vi "UHR-Fleezers Control (host) - Lorentz v5.vi"() -> ()   [LabVIEW 2014] (continued)
                n1783 = Number To Decimal String(number="Flush rate (uL/m)") -> (decimal integer string=w2729:string)  [unwired: 1 in]
                n1784 = Concatenate Strings("irate  " ("string"), w2729, " u/m" ("string"), "\r") -> (w2731:string)
                n1785 = VISA Write(VISA resource name=w2733, write buffer=w2731) -> (VISA resource name out=w2727:refnum<visa-resource-name>)  [unwired: 1 in, 2 out]
                n1786 = Reciprocal(x="Flush rate (uL/m)") -> (1/x=w2712:dbl)
                n1787 = Number To Decimal String(number="Volume (uL)") -> (decimal integer string=w2718:string)  [unwired: 1 in]
                n1788 = Multiply(x="Volume (uL)", y=w2712) -> (x*y=w2711:dbl)
                n1789 = Concatenate Strings("tvolume  " ("string"), w2718, " u" ("string"), "\r") -> (w2716:string)
                n1790 = Multiply(x=w2711, y=60000.0) -> (x*y=w2709:dbl)
                n1791 = VISA Write(VISA resource name=w2727, write buffer=w2716) -> (VISA resource name out=w2715:refnum<visa-resource-name>)  [unwired: 1 in, 2 out]
                n1792 = Concatenate Strings("cvolume" ("string"), "\r") -> (w2714:string)
                n1793 = VISA Write(VISA resource name=w2715, write buffer=w2714) -> (VISA resource name out=w2725:refnum<visa-resource-name>)  [unwired: 1 in, 2 out]
                n1794 = Concatenate Strings("irun" ("string"), "\r") -> (w2723:string)
                n1795 = VISA Write(VISA resource name=w2725, write buffer=w2723) -> (VISA resource name out=w2713:refnum<visa-resource-name>)  [unwired: 1 in, 2 out]
              }
              frame #1 {
                # "Have to wait until\nflow is done to reset\nrate"
                n1796 = Add(x=w2736, y=100.0) -> (x+y=w2735:dbl)
                n1797 = Wait (ms)(milliseconds to wait=w2735) -> ()  [unwired: 1 out]
              }
              frame #2 {
                # "reset flow rate to usual flow rate"
                n1798 = local read "Flow rate (uL/h)"() -> (w2748:dbl)
                n1799 = Number To Decimal String(number=w2748) -> (decimal integer string=w2746:string)  [unwired: 1 in]
                n1800 = Concatenate Strings("irate  " ("string"), w2746, " u/h" ("string"), "\r") -> (w2744:string)
                n1801 = VISA Write(VISA resource name=w2742, write buffer=w2744) -> (VISA resource name out=w2738:refnum<visa-resource-name>)  [unwired: 1 in, 2 out]
                n1802 = Concatenate Strings("cvolume" ("string"), "\r") -> (w2739:string)
                n1803 = VISA Write(VISA resource name=w2738, write buffer=w2739) -> ()  [unwired: 1 in, 3 out]
              }
            }
            n1804 = local read "Save Event Log?"() -> (w2688:bool)
            n1805 = local read "Saving..."() -> (w2687:bool)
            n1806 = And(x=w2688, y=w2687) -> (x .and. y?=w2689:bool)
            n1807 = case shown="True" w2689 {
              tunnel: w2691 -> [_ w2698]
              tunnel: w2690 -> [_ w2697]
              frame False {
              }
              frame True {
                n1808 = Number To Decimal String(number=w2698) -> (decimal integer string=w2702:string)  [unwired: 1 in]
                n1809 = Number To Decimal String(number=w2697) -> (decimal integer string=w2704:string)  [unwired: 1 in]
                n1810 = local read "log file ref"() -> (w2699:refnum<file>)
                n1811 = local read "Time (s)"() -> (w2700:dbl)
                n1812 = Concatenate Strings("pump 2 flushing ", w2702, " uL at ", w2704, " ul/min") -> (w2706:string)
                n1813 = call "write to event log.vi"("log file ref"=w2699, "time"=w2700, "input string"=w2706) -> ()  [unwired: 8 in]
              }
            }
          }
          frame Enabled {
          }
        }
      }
      event "Flush Pump 3": Value Change {
        n1814 = event-data() -> ()  [unwired: 7 out]
        n1815 = disable-structure shown="Disabled" {
          disable-tunnel: ["Flush Pump 3" _] -> w2750
          disable-tunnel: w2749 -> [w2756 _]
          frame Disabled {
            n1816 = flat-sequence {
              tunnel: w2756 -> [w2771]
              tunnel: ["Flush rate (uL/m) P3"] -> w2752
              tunnel: ["Volume (uL) P3"] -> w2751
              frame #0 {
                # "set paramaters (rate, volume) for flush, clear volume"
                n1817 = Number To Decimal String(number="Flush rate (uL/m) P3") -> (decimal integer string=w2791:string)  [unwired: 1 in]
                n1818 = local write "Inject Pump 3"(TRUE ("Inject Pump 3")) -> ()
                n1819 = Concatenate Strings("irate  " ("string"), w2791, " u/m" ("string"), "\r") -> (w2793:string)
                n1820 = VISA Write(VISA resource name=w2771, write buffer=w2793) -> (VISA resource name out=w2789:refnum<visa-resource-name>)  [unwired: 1 in, 2 out]
                n1821 = Reciprocal(x="Flush rate (uL/m) P3") -> (1/x=w2775:dbl)
                n1822 = Number To Decimal String(number="Volume (uL) P3") -> (decimal integer string=w2780:string)  [unwired: 1 in]
                n1823 = Multiply(x="Volume (uL) P3", y=w2775) -> (x*y=w2774:dbl)
                n1824 = Concatenate Strings("tvolume  " ("string"), w2780, " u" ("string"), "\r") -> (w2778:string)
                n1825 = Multiply(x=w2774, y=60.0) -> (x*y=→"HP3 Flush Time (s)":dbl)
                n1826 = VISA Write(VISA resource name=w2789, write buffer=w2778) -> (VISA resource name out=w2777:refnum<visa-resource-name>)  [unwired: 1 in, 2 out]
                n1827 = Concatenate Strings("cvolume" ("string"), "\r") -> (w2776:string)
                n1828 = VISA Write(VISA resource name=w2777, write buffer=w2776) -> (VISA resource name out=w2787:refnum<visa-resource-name>)  [unwired: 1 in, 2 out]
                n1829 = Concatenate Strings("irun" ("string"), "\r") -> (w2785:string)
                n1830 = VISA Write(VISA resource name=w2787, write buffer=w2785) -> ()  [unwired: 1 in, 3 out]
              }
              frame #1 {
                "Flushing P3" <- TRUE ("Flushing P3")
              }
            }
            n1831 = local read "Save Event Log?"() -> (w2754:bool)
            n1832 = local read "Saving..."() -> (w2755:bool)
            n1833 = And(x=w2754, y=w2755) -> (x .and. y?=w2753:bool)
            n1834 = case shown="True" w2753 {
              tunnel: w2752 -> [_ w2759]
              tunnel: w2751 -> [_ w2758]
              frame False {
              }
              frame True {
                n1835 = Number To Decimal String(number=w2758) -> (decimal integer string=w2763:string)  [unwired: 1 in]
                n1836 = Number To Decimal String(number=w2759) -> (decimal integer string=w2765:string)  [unwired: 1 in]
                n1837 = local read "log file ref"() -> (w2760:refnum<file>)
                n1838 = local read "Time (s)"() -> (w2761:dbl)
                n1839 = Concatenate Strings("pump 3 flushing ", w2763, " uL at ", w2765, " ul/min") -> (w2767:string)
                n1840 = call "write to event log.vi"("log file ref"=w2760, "time"=w2761, "input string"=w2767) -> ()  [unwired: 8 in]
              }
            }
          }
          frame Enabled {
          }
        }
      }
      event "Flush Pump 1": Value Change {
        n1841 = event-data() -> ()  [unwired: 7 out]
        n1842 = disable-structure shown="Disabled" {
          disable-tunnel: ["Flush Pump 1" _] -> w2797
          disable-tunnel: w2796 -> [w2803 _]
          frame Disabled {
            n1843 = flat-sequence {
              tunnel: [w2824] -> w2805
              tunnel: w2803 -> [w2819]
              tunnel: ["Volume (uL) P1"] -> w2799
              tunnel: ["Flush rate (uL/m) P1"] -> w2798
              tunnel: w2805 -> [_]
              frame #0 {
                # "set paramaters (rate, volume) for flush, clear volume"
                n1844 = local write "Inject Pump 1"(TRUE ("Inject Pump 1")) -> ()
                n1845 = Number To Decimal String(number="Flush rate (uL/m) P1") -> (decimal integer string=w2840:string)  [unwired: 1 in]
                n1846 = Concatenate Strings("irate  " ("string"), w2840, " u/m" ("string"), "\r") -> (w2842:string)
                n1847 = VISA Write(VISA resource name=w2819, write buffer=w2842) -> (VISA resource name out=w2838:refnum<visa-resource-name>)  [unwired: 1 in, 2 out]
                n1848 = Reciprocal(x="Flush rate (uL/m) P1") -> (1/x=w2823:dbl)
                n1849 = Number To Decimal String(number="Volume (uL) P1") -> (decimal integer string=w2829:string)  [unwired: 1 in]
                n1850 = Multiply(x="Volume (uL) P1", y=w2823) -> (x*y=w2822:dbl)
                n1851 = Concatenate Strings("tvolume  " ("string"), w2829, " u" ("string"), "\r") -> (w2827:string)
                n1852 = Multiply(x=w2822, y=60.0) -> (x*y=→"HP1 Flush Time (s)":dbl)
                n1853 = VISA Write(VISA resource name=w2838, write buffer=w2827) -> (VISA resource name out=w2826:refnum<visa-resource-name>)  [unwired: 1 in, 2 out]
                n1854 = Concatenate Strings("cvolume" ("string"), "\r") -> (w2825:string)
                n1855 = VISA Write(VISA resource name=w2826, write buffer=w2825) -> (VISA resource name out=w2836:refnum<visa-resource-name>)  [unwired: 1 in, 2 out]
                n1856 = Concatenate Strings("irun" ("string"), "\r") -> (w2834:string)
                n1857 = VISA Write(VISA resource name=w2836, write buffer=w2834) -> (VISA resource name out=w2824:refnum<visa-resource-name>)  [unwired: 1 in, 2 out]
              }
              frame #1 {
                "Flushing P1" <- TRUE ("Flushing P3")
              }
            }
            n1858 = local read "Saving..."() -> (w2800:bool)
            n1859 = local read "Save Event Log?"() -> (w2801:bool)
            n1860 = And(x=w2801, y=w2800) -> (x .and. y?=w2802:bool)
            n1861 = case shown="True" w2802 {
              tunnel: w2799 -> [_ w2808]
              tunnel: w2798 -> [_ w2807]
              frame False {
              }
              frame True {
                n1862 = Number To Decimal String(number=w2808) -> (decimal integer string=w2812:string)  [unwired: 1 in]
                n1863 = Number To Decimal String(number=w2807) -> (decimal integer string=w2810:string)  [unwired: 1 in]
                n1864 = local read "log file ref"() -> (w2814:refnum<file>)
                n1865 = local read "Time (s)"() -> (w2815:dbl)
                n1866 = Concatenate Strings("pump 1 flushing ", w2812, " uL at ", w2810, " ul/min") -> (w2806:string)
                n1867 = call "write to event log.vi"("log file ref"=w2814, "time"=w2815, "input string"=w2806) -> ()  [unwired: 8 in]
              }
            }
          }
          frame Enabled {
          }
        }
      }
      event "Clear Volume": Value Change {
        n1868 = event-data() -> ()  [unwired: 7 out]
        n1869 = disable-structure shown="Disabled" {
          disable-tunnel: ["Clear Volume" _] -> w2846
          disable-tunnel: w2845 -> [w2847 _]
          frame Disabled {
            n1870 = Concatenate Strings("cvolume" ("string"), "\r") -> (w2848:string)
            n1871 = VISA Write(VISA resource name=w2847, write buffer=w2848) -> ()  [unwired: 1 in, 3 out]
          }
          frame Enabled {
          }
        }
      }
      event "Clear Volume P3": Value Change {
        n1872 = event-data() -> ()  [unwired: 7 out]
        n1873 = disable-structure shown="Disabled" {
          disable-tunnel: w2852 -> [w2854 _]
          frame Disabled {
            n1874 = Concatenate Strings("cvolume" ("string"), "\r") -> (w2855:string)
            n1875 = VISA Write(VISA resource name=w2854, write buffer=w2855) -> ()  [unwired: 1 in, 3 out]
            n1876 = local write "Clear Volume P3"(FALSE ("Clear Volume P3")) -> ()
          }
          frame Enabled {
          }
        }
      }
      event "Clear Volume P1": Value Change {
        n1877 = event-data() -> ()  [unwired: 7 out]
        n1878 = disable-structure shown="Disabled" {
          disable-tunnel: w2858 -> [w2860 _]
          frame Disabled {
            n1879 = Concatenate Strings("cvolume" ("string"), "\r") -> (w2861:string)
            n1880 = local write "Clear Volume P1"(FALSE ("Clear Volume P1")) -> ()
            n1881 = VISA Write(VISA resource name=w2860, write buffer=w2861) -> ()  [unwired: 1 in, 3 out]
          }
          frame Enabled {
          }
        }
      }
      event "Display On P3": Value Change {
        n1882 = event-data() -> ()  [unwired: 7 out]
        n1883 = disable-structure shown="Disabled" {
          disable-tunnel: w2864 -> [w2865 _]
          frame Disabled {
            n1884 = Select(t="dim 100", s="Display On P3", f="dim 0") -> (s? t:f=w2868:string)
            n1885 = Concatenate Strings(w2868, "\r") -> (w2870:string)
            n1886 = VISA Write(VISA resource name=w2865, write buffer=w2870) -> ()  [unwired: 1 in, 3 out]
          }
          frame Enabled {
          }
        }
      }
      event "Display On P1": Value Change {
        n1887 = event-data() -> ()  [unwired: 7 out]
        n1888 = disable-structure shown="Disabled" {
          disable-tunnel: w2872 -> [w2873 _]
          frame Disabled {
            n1889 = Select(t="dim 100", s="Display On P1", f="dim 0") -> (s? t:f=w2876:string)
            n1890 = Concatenate Strings(w2876, "\r") -> (w2878:string)
            n1891 = VISA Write(VISA resource name=w2873, write buffer=w2878) -> ()  [unwired: 1 in, 3 out]
          }
          frame Enabled {
          }
        }
      }
      event "Retract Pump 3": Value Change {
        n1892 = event-data() -> ()  [unwired: 7 out]
        n1893 = disable-structure shown="Disabled" {
          disable-tunnel: w2880 -> [w2881 _]
          frame Disabled {
            n1894 = local write "Retract Pump 3"(FALSE ("Retract Pump 3")) -> ()
            n1895 = case shown="True" "Retract Pump 3" {
              tunnel: w2881 -> [_ w2884]
              frame False {
              }
              frame True {
                n1896 = Number To Decimal String(number="Retract Rate (uL/m)") -> (decimal integer string=w2902:string)  [unwired: 1 in]
                n1897 = Concatenate Strings("wrate  " ("string"), w2902, " u/m" ("string"), "\r") -> (w2904:string)
                n1898 = VISA Write(VISA resource name=w2884, write buffer=w2904) -> (VISA resource name out=w2895:refnum<visa-resource-name>)  [unwired: 1 in, 2 out]
                n1899 = Number To Decimal String(number="Retract Vol 3 (uL)") -> (decimal integer string=w2897:string)  [unwired: 1 in]
                n1900 = Concatenate Strings("tvolume  " ("string"), w2897, " u" ("string"), "\r") -> (w2894:string)
                n1901 = VISA Write(VISA resource name=w2895, write buffer=w2894) -> (VISA resource name out=w2890:refnum<visa-resource-name>)  [unwired: 1 in, 2 out]
                n1902 = Concatenate Strings("cvolume" ("string"), "\r") -> (w2891:string)
                n1903 = VISA Write(VISA resource name=w2890, write buffer=w2891) -> (VISA resource name out=w2885:refnum<visa-resource-name>)  [unwired: 1 in, 2 out]
                n1904 = Concatenate Strings("wrun" ("string"), "\r") -> (w2886:string)
                n1905 = VISA Write(VISA resource name=w2885, write buffer=w2886) -> ()  [unwired: 1 in, 3 out]
              }
            }
          }
          frame Enabled {
          }
        }
      }
      event "Retract Pump 1": Value Change {
        n1906 = event-data() -> ()  [unwired: 7 out]
        n1907 = disable-structure shown="Disabled" {
          disable-tunnel: w2906 -> [w2907 _]
          frame Disabled {
            n1908 = local write "Retract Pump 1"(FALSE ("Retract Pump 1")) -> ()
            n1909 = case shown="True" "Retract Pump 1" {
              tunnel: w2907 -> [_ w2912]
              frame False {
              }
              frame True {
                n1910 = local read "Retract Rate (uL/m)"() -> (w2910:dbl)
                n1911 = Number To Decimal String(number=w2910) -> (decimal integer string=w2928:string)  [unwired: 1 in]
                n1912 = Concatenate Strings("wrate  " ("string"), w2928, " u/m" ("string"), "\r") -> (w2930:string)
                n1913 = VISA Write(VISA resource name=w2912, write buffer=w2930) -> (VISA resource name out=w2922:refnum<visa-resource-name>)  [unwired: 1 in, 2 out]
                n1914 = Number To Decimal String(number="Retract Vol 1 (uL)") -> (decimal integer string=w2924:string)  [unwired: 1 in]
                n1915 = Concatenate Strings("tvolume  " ("string"), w2924, " u" ("string"), "\r") -> (w2921:string)
                n1916 = VISA Write(VISA resource name=w2922, write buffer=w2921) -> (VISA resource name out=w2918:refnum<visa-resource-name>)  [unwired: 1 in, 2 out]
                n1917 = Concatenate Strings("cvolume" ("string"), "\r") -> (w2919:string)
                n1918 = VISA Write(VISA resource name=w2918, write buffer=w2919) -> (VISA resource name out=w2913:refnum<visa-resource-name>)  [unwired: 1 in, 2 out]
                n1919 = Concatenate Strings("wrun" ("string"), "\r") -> (w2914:string)
                n1920 = VISA Write(VISA resource name=w2913, write buffer=w2914) -> ()  [unwired: 1 in, 3 out]
              }
            }
          }
          frame Enabled {
          }
        }
      }
      event "Flip Green Filter": Value Change {
        n1921 = event-data() -> ()  [unwired: 7 out]
        n1922 = Not(x="Flip Green Filter") -> (.not. x?=w2933:bool)
        n1923 = local write "Flip Green Filter"(w2933) -> ()
        n1924 = flat-sequence {
          tunnel: [w2942] -> w2938
          tunnel: [w2941] -> w2937
          tunnel: w2932 -> [w2940]
          tunnel: [w2945] -> w2936
          tunnel: w2938 -> [w2945]
          tunnel: [w2944] -> w2935
          tunnel: w2937 -> [w2944]
          tunnel: w2936 -> [w2949]
          tunnel: w2935 -> [w2948]
          tunnel: [w2947] -> w2939
          frame #0 {
            n1925 = xnode "Read/Write Control"("FPGA VI Reference In"=w2940, "Green Filter Flipper"=TRUE) -> ("FPGA VI Reference Out"=w2942:T35, "error out"=w2941:errorcluster)  [unwired: 1 in]
          }
          frame #1 {
            n1926 = Wait (ms)(milliseconds to wait=u32 100) -> ()  [unwired: 1 out]
          }
          frame #2 {
            n1927 = xnode "Read/Write Control"("FPGA VI Reference In"=w2949, "error in"=w2948, "Green Filter Flipper"=FALSE) -> ("error out"=w2947:errorcluster)  [unwired: 1 out]
          }
        }
      }
      event "Pump 1 contents", "Pump 3 contents": Value Change {
        n1928 = event-data() -> ()  [unwired: 7 out]
        n1929 = local read "Pump 1 contents"() -> (→"Pump 1 cont disp":string)
        n1930 = local read "Pump 3 contents"() -> (→"Pump 3 cont disp":string)
      }
      event "Reset Trap Pos. FB": Value Change {
        n1931 = event-data() -> ()  [unwired: 7 out]
        n1932 = xnode "Read/Write Control"("FPGA VI Reference In"=w2953, "Trap Pos. FB Reset"="Reset Trap Pos. FB") -> ()  [unwired: 1 in, 2 out]
      }
      event "Rem fb disp offset": Value Change {
        n1933 = event-data() -> ()  [unwired: 7 out]
        n1934 = local write "Rem fb disp offset"(FALSE ("Rem fb disp offset")) -> ()
        n1935 = local read "Mean Trap Positions (nm)"() -> (w2956:T4)
        n1936 = local read "FB Trap Pos Offset"() -> (w2958:dbl)
        n1937 = Unbundle By Name(w2956) -> ("T1 X"=w2955:dbl)
        n1938 = Subtract(x=w2958, y=w2955) -> (x-y=w2957:dbl)
        n1939 = local write "FB Trap Pos Offset"(w2957) -> ()
      }
      event "Threshold (nm)": Value Change {
        n1940 = event-data() -> ()  [unwired: 7 out]
        n1941 = flat-sequence {
          tunnel: [w2963] -> w2961
          tunnel: w2960 -> [w2962]
          tunnel: w2961 -> [w2974]
          frame #0 {
            n1942 = xnode "Read/Write Control"("FPGA VI Reference In"=w2962) -> ("FPGA VI Reference Out"=w2966:T35, "error out"=w2965:errorcluster, "FPGA TTrig Thresh"=w2967:i64)  [unwired: 1 in]
            n1943 = local read "Threshold stored (nm)"() -> (w2973:dbl)
            n1944 = local read "Threshold (nm)"() -> (w2963:dbl)
            n1945 = local read "AOM X Cal (nm/MHz)"() -> (w2971:dbl)
            n1946 = Subtract(x=w2963, y=w2973) -> (x-y=w2972:dbl)
            n1947 = Divide(x=w2972, y=w2971) -> (x/y=w2969:dbl)
            n1948 = call "IR AOM freq to word.vi"("Frequency In (MHz)"=w2969) -> ("Frequency Word Out (double)"=w2970:dbl)
            n1949 = To Quad Integer(1:w2970) -> (0:w2968:i64)
            n1950 = Add(x=w2967, y=w2968) -> (x+y=w2964:i64)
            n1951 = xnode "Read/Write Control"("FPGA VI Reference In"=w2966, "error in"=w2965, "FPGA TTrig Thresh"=w2964) -> ()  [unwired: 2 out]
          }
          frame #1 {
            "Threshold stored (nm)" <- w2974
          }
        }
      }
      event "FB Trig Integrate": Value Change {
        n1952 = event-data() -> ()  [unwired: 7 out]
        n1953 = local read "FB Trig Integrate"() -> (w2977:u32)
        n1954 = xnode "Read/Write Control"("FPGA VI Reference In"=w2975, "FB Trig Integrate"=w2977) -> ("error out"=w2976:errorcluster)  [unwired: 1 in, 1 out]
      }
      event "11": Value Change {
        n1955 = event-data() -> ()  [unwired: 7 out]
        n1956 = local read "11"() -> (w2978:bool)
        n1957 = case shown="True" w2978 {
          frame False {
          }
          frame True {
            n1958 = local read "Messages"() -> (w2980:string)
            n1959 = call "Update messages.vi"("Message to add"="You kicked it up to 11!", "Old message string"=w2980) -> ("New message string"=w2981:string)
            n1960 = call <vilib>:"Beep.vi"() -> ()  [unwired: 12 in]
            n1961 = local write "Messages"(w2981) -> ()
          }
        }
      }
      event "Trap Pos. FB ON": Value Change {
        w2988 = 6.0  # clock mult.
        w2987 = 49152000.0  # TCXO frequ.
        n1962 = event-data() -> ()  [unwired: 7 out]
        n1963 = xnode "Read/Write Control"("FPGA VI Reference In"=w2982) -> ("FPGA VI Reference Out"=w2984:T35, "BD1 Frequency Out 1"=w2985:u64)  [unwired: 1 in, 1 out]
        n1964 = To Double Precision Float(number=w2985) -> (double precision float=w2989:dbl)
        n1965 = Multiply(x=w2987, y=w2988) -> (x*y=w2990:dbl)
        n1966 = Multiply(x=w2989, y=w2990) -> (x*y=w2991:dbl)
        n1967 = Scale By Power Of 2(n=-48, x=w2991) -> (x*2^n=w2993:dbl)
        n1968 = Divide(x=w2993, y=1000000.0) -> (x/y=w2986:dbl)
        n1969 = flat-sequence {
          tunnel: w2984 -> [w2999]
          tunnel: [w2998] -> w2995
          tunnel: "Trap Pos. FB ON" -> [w2997]
          tunnel: w2985 -> [w2996]
          tunnel: w2995 -> [w3005]
          tunnel: "Trap Pos. FB ON" -> [w3004]
          tunnel: w2986 -> [w3007]
          tunnel: "Trap Pos. FB ON" -> [w3006]
          frame #0 {
            n1970 = case shown="False" w2997 {
              tunnel: w2999 -> [w3001 w3003]
              tunnel: [w3002 w3003] -> w2998
              tunnel: w2996 -> [w3000 _]
              frame False {
                n1971 = xnode "Read/Write Control"("FPGA VI Reference In"=w3001, "BD 1 Frequency 1"=w3000) -> ("FPGA VI Reference Out"=w3002:T35)  [unwired: 1 in, 1 out]
              }
              frame True {
              }
            }
          }
          frame #1 {
            n1972 = xnode "Read/Write Control"("FPGA VI Reference In"=w3005, "Force feedback"=w3004) -> ()  [unwired: 1 in, 2 out]
          }
          frame #2 {
            n1973 = case shown="False" w3006 {
              tunnel: w3007 -> [w3008 _]
              frame False {
                n1974 = property on="BD 1 Frequency 1 (MHz)" class="DigNum (strict)"("Val(Sgnl)"=w3008) -> ()  [unwired: 2 in, 2 out]
              }
              frame True {
              }
            }
          }
        }
      }
      event "Remove Action Offset": Value Change {
        n1975 = event-data() -> ()  [unwired: 7 out]
        n1976 = local write "Remove Action Offset"(FALSE ("Remove Action Offset")) -> ()
        n1977 = local read "Trap Pos. FB Mult Factor"() -> (w3014:i64)
        n1978 = local read "Trap Pos FB Action"() -> (w3012:i64)
        n1979 = local read "Trap Pos. FB Offset Factor"() -> (w3010:i64)
        n1980 = Multiply(x=w3014, y=w3012) -> (x*y=w3013:i64)
        n1981 = Add(x=w3013, y=w3010) -> (x+y=w3011:i64)
        n1982 = local write "Trap Pos. FB Offset Factor"(w3011) -> ()
        n1983 = xnode "Read/Write Control"("FPGA VI Reference In"=w3009, "Trap Pos. FB Offset Factor"=w3011) -> ()  [unwired: 1 in, 2 out]
      }
      event "Remove Unwinding Offset": Value Change {
        n1984 = event-data() -> ()  [unwired: 7 out]
        n1985 = local write "Remove Unwinding Offset"(FALSE ("Remove Action Offset")) -> ()
        n1986 = local read "Trap Pos. FB Mult Factor"() -> (w3028:i64)
        n1987 = local read "Trap Pos FB Action"() -> (w3026:i64)
        n1988 = local read "Trap Pos. FB Offset Factor"() -> (w3025:i64)
        n1989 = Multiply(x=w3028, y=w3026) -> (x*y=w3027:i64)
        n1990 = local read "Trap Pos. FB Mult Factor"() -> (w3024:i64)
        n1991 = Add(x=w3027, y=w3025) -> (x+y=w3018:i64)
        n1992 = Multiply(x=32768, y="factor") -> (x*y=w3021:dbl)
        n1993 = Multiply(x=w3021, y=w3024) -> (x*y=w3023:dbl)
        n1994 = Subtract(x=w3018, y=w3023) -> (x-y=w3022:dbl)
        n1995 = To Quad Integer(1:w3022) -> (0:w3017:i64)
        n1996 = xnode "Read/Write Control"("FPGA VI Reference In"=w3016, "Trap Pos. FB Offset Factor"=w3017) -> ()  [unwired: 1 in, 2 out]
        n1997 = local write "Trap Pos. FB Offset Factor"(w3017) -> ()
      }
      event "Trap Pos. FB Range", "Trap Pos. FB Gains", "Trap Pos. FB Mult Factor", "Trap Pos. FB Offset Factor", "Trap Pos FB Negate Action", "Trap Pos FB Monitor\nT1 or T2", "Differential FB?", "Negate Diff?": Value Change {
        n1998 = event-data() -> ()  [unwired: 7 out]
        n1999 = local read "Negate Diff?"() -> (w3033:bool)
        n2000 = xnode "Read/Write Control"("FPGA VI Reference In"=w3032, "Trap Pos. FB Gains"="Trap Pos. FB Gains", "Trap pos. FB Range"="Trap Pos. FB Range", "Trap Pos. FB Mult Factor"="Trap Pos. FB Mult Factor", "Trap Pos. FB Offset Factor"="Trap Pos. FB Offset Factor", "Trap Pos FB Negate Action"="Trap Pos FB Negate Action", "Trap Pos FB Monitor T1 or T2"="Trap Pos FB Monitor\nT1 or T2", "AI1 X Scale"="Trap Pos. AI1 X Pre-scale", "Negate Diff?"=w3033, "Diff FB Measurement?"="Differential FB?") -> ()  [unwired: 1 in, 2 out]
      }
      event "Trap Pos FB SP", "Trap Pos FB SP 2", "Use SP 2": Value Change {
        n2001 = event-data() -> ()  [unwired: 7 out]
        n2002 = Select(t="Trap Pos FB SP 2", s="Use SP 2", f="Trap Pos FB SP") -> (s? t:f=w3041:fxp<+/-,16,1>)
        n2003 = xnode "Read/Write Control"("FPGA VI Reference In"=w3040, "Trap Pos. FB SP"=w3041) -> ()  [unwired: 1 in, 2 out]
      }
      event "Offset SP2 from SP1": Value Change {
        n2004 = event-data() -> ()  [unwired: 7 out]
        n2005 = local read "Trap Pos FB SP"() -> (w3047:fxp<+/-,16,1>)
        n2006 = Add(x=w3047, y="SP2 Offset") -> (x+y=w3045:fxp<+/-,16,1>)
        n2007 = property on="Trap Pos FB SP 2" class="DigNum (strict)"("Val(Sgnl)"=w3045) -> ()  [unwired: 2 in, 2 out]
        n2008 = local write "Offset SP2 from SP1"(FALSE ("Offset SP2 from SP1")) -> ()
      }
      event "Set Reading to\nSetpoint": Value Change {
        # "This is the actual PID input signal"
        n2009 = event-data() -> ()  [unwired: 7 out]
        n2010 = local write "Set Reading to\nSetpoint"(FALSE ("Set SP to Reading")) -> ()
        n2011 = xnode "Read/Write Control"("FPGA VI Reference In"=w3051) -> ("FPGA VI Reference Out"=w3054:T35, "error out"=w3053:errorcluster, "Trap Pos FB Int-Norm Signal"=w3052:fxp<+/-,16,1>, "BD1 Frequency Out 1"=w3050:u64)  [unwired: 1 in]
        n2012 = local read "Differential FB?"() -> (w3055:bool)
        n2013 = case shown="False" w3055 {
          tunnel: [w3084 w3091] -> w3049
          tunnel: w3052 -> [w3082 w3091]
          frame False {
            n2014 = local read "Trap Pos FB Monitor\nT1 or T2"() -> (w3087:bool)
            n2015 = local read "Trap X AI1 (DMA)"() -> (w3090:T19)
            n2016 = Unbundle By Name(w3090) -> ("Set 1"=w3089:fxp<+/-,16,1>, "Set 2"=w3088:fxp<+/-,16,1>)
            n2017 = Select(t=w3089, s=w3087, f=w3088) -> (s? t:f=w3086:fxp<+/-,16,1>)
            n2018 = Not(x="Set SP Using...") -> (.not. x?=w3083:bool)
            n2019 = Select(t=w3082, s=w3083, f=w3086) -> (s? t:f=w3084:fxp<+/-,16,1>)
          }
          frame True {
          }
        }
        n2020 = disable-structure shown="Disabled" {
          disable-tunnel: _ -> [w3060 _]
          disable-tunnel: w3050 -> [w3059 _]
          disable-tunnel: w3049 -> [w3058 _]
          frame Disabled {
            n2021 = case shown="True" w3060 {
              tunnel: [w3061 w3063] -> w3057
              tunnel: w3058 -> [w3061 w3062]
              tunnel: w3059 -> [_ w3081]
              frame False {
              }
              frame True {
                w3079 = 6.0  # clock mult.
                w3080 = 49152000.0  # TCXO frequ.
                # "Added by Ronen - for the real time\nchange of the setpoint to accomodate \nchanges in the offset."
                n2022 = To Double Precision Float(number=w3081) -> (double precision float=w3078:dbl)
                n2023 = local read "BD 1 Frequency 2 (MHz)"() -> (w3071:dbl)
                n2024 = Multiply(x=w3080, y=w3079) -> (x*y=w3077:dbl)
                n2025 = Multiply(x=w3078, y=w3077) -> (x*y=w3076:dbl)
                n2026 = local read "Offset file step size"() -> (w3069:dbl)
                n2027 = Scale By Power Of 2(n=-48, x=w3076) -> (x*2^n=w3074:dbl)
                n2028 = Divide(x=w3074, y=1000000.0) -> (x/y=w3072:dbl)
                n2029 = Subtract(x=w3071, y=w3072) -> (x-y=w3070:dbl)
                n2030 = Divide(x=w3070, y=w3069) -> (x/y=w3068:dbl)
                n2031 = local read item#-1() -> (w3066)
                n2032 = To Long Integer(number=w3068) -> (32bit integer=w3067:i32)
                n2033 = Index Array(array=w3066, index=w3067) -> (element=w3065)
                n2034 = To Fixed-Point(number=w3065) -> (fixed-point=w3064:fxp<+/-,16,1>)  [unwired: 1 in]
                n2035 = Add(x=w3062, y=w3064) -> (x+y=w3063:fxp<+/-,17,2>)
              }
            }
            "Offset corrected setpoint" <- w3057
          }
          frame Enabled {
          }
        }
        n2036 = local write "Trap Pos FB SP"(w3049) -> ()
        n2037 = xnode "Read/Write Control"("FPGA VI Reference In"=w3054, "error in"=w3053, "Trap Pos. FB SP"=w3049) -> ()  [unwired: 2 out]
      }
      event "Trap Pos. FB Out Scale 2^n": Value Change {
        n2038 = event-data() -> ()  [unwired: 7 out]
        n2039 = Scale By Power Of 2(n="Trap Pos. FB Out Scale 2^n", x=ext 1.0) -> (x*2^n=w3092:ext)
        n2040 = property on="Trap Pos. FB Mult Factor" class="DigNum (strict)"("Val(Sgnl)"=w3092) -> ()  [unwired: 2 in, 2 out]
      }
      event "Trap Pos FB Int Count": Value Change {
        n2041 = event-data() -> ()  [unwired: 7 out]
        n2042 = xnode "Read/Write Control"("FPGA VI Reference In"=w3095, "Trap Pos FB Int Count"="Trap Pos FB Int Count") -> ()  [unwired: 1 in, 2 out]
      }
      event "Display Saved Data": Value Change {
        n2043 = event-data() -> ()  [unwired: 7 out]
        n2044 = case shown="\"Amp Current\"" "Display Saved Data" {
          frame "Bead Seperation", Default {
            n2045 = property on="Amp current" class="WFGraph (strict)"("Visible"=FALSE) -> ()  [unwired: 2 in, 2 out]
            n2046 = property on="Trap Delta Graph" class="WFGraph (strict)"("Visible"=TRUE) -> ()  [unwired: 2 in, 2 out]
            n2047 = property on="Saved trap pos" class="WFGraph (strict)"("Visible"=FALSE) -> ()  [unwired: 2 in, 2 out]
          }
          frame "Amp Current" {
            n2048 = property on="Saved trap pos" class="WFGraph (strict)"("Visible"=FALSE) -> ()  [unwired: 2 in, 2 out]
            n2049 = property on="Trap Delta Graph" class="WFGraph (strict)"("Visible"=FALSE) -> ()  [unwired: 2 in, 2 out]
            n2050 = property on="Amp current" class="WFGraph (strict)"("Visible"=TRUE) -> ()  [unwired: 2 in, 2 out]
          }
          frame "Trap Position" {
            n2051 = property on="Saved trap pos" class="WFGraph (strict)"("Visible"=TRUE) -> ()  [unwired: 2 in, 2 out]
            n2052 = property on="Trap Delta Graph" class="WFGraph (strict)"("Visible"=FALSE) -> ()  [unwired: 2 in, 2 out]
            n2053 = property on="Amp current" class="WFGraph (strict)"("Visible"=FALSE) -> ()  [unwired: 2 in, 2 out]
          }
        }
      }
      event "Calibration": Value Change {
        n2054 = event-data() -> ()  [unwired: 7 out]
        n2055 = local read "X or Y?"() -> (w3123:bool)
        n2056 = local read "Calibration"() -> (w3120:u16)
        n2057 = Select(t="X" ("Label.Text"), s=w3123, f="Y" ("Label.Text")) -> (s? t:f=w3117:string)
        n2058 = case shown="0, Default" w3120 {
          tunnel: ["Position (V)" ("Label.Text") "Position (nm)" ("Label.Text") "Force (pN)" ("Label.Text")] -> w3114
          tunnel: [" (V)" ("Label.Text") " (nm)" ("Label.Text") " (pN)" ("Label.Text")] -> w3111
          frame 0, Default {
          }
          frame 1 {
          }
          frame 2 {
          }
        }
        n2059 = Concatenate Strings("T1 " ("Label.Text"), w3117) -> (w3113:string)
        n2060 = Concatenate Strings("T2 " ("Label.Text"), w3117) -> (w3112:string)
        n2061 = property on="Force" class="WFChart (strict)"("YScale.NameLbl.Text"=w3114) -> ()  [unwired: 2 in, 2 out]
        n2062 = Concatenate Strings("Mean" ("Label.Text"), w3111) -> (w3110:string)
        n2063 = Concatenate Strings(w3113, w3111) -> (w3109:string)
        n2064 = Concatenate Strings(w3112, w3111) -> (w3108:string)
        n2065 = Concatenate Strings("Difference" ("Label.Text"), w3111) -> (w3107:string)
        n2066 = property on="Mean" class="DigNum (strict)"("Caption.Text"=w3110) -> ()  [unwired: 2 in, 2 out]
        n2067 = property on="T1 X" class="DigNum (strict)"("Caption.Text"=w3109) -> ()  [unwired: 2 in, 2 out]
        n2068 = property on="T2 X" class="DigNum (strict)"("Caption.Text"=w3108) -> ()  [unwired: 2 in, 2 out]
        n2069 = property on="Difference" class="DigNum (strict)"("Caption.Text"=w3107) -> ()  [unwired: 2 in, 2 out]
      }
      event "Base N trap periods", "Period scale factor", "Trap osc amp (MHz)", "Cal sets to save", "# Samples/trap", "Total Counts (ticks)": Value Change {
        w3130 = 1.0
        w3136 = u32 0 ("y")
        # "scales 0 to 2pi"
        # "Create vector of trap offset (oscillation) values."
        # "Compute oscillation period as a multiple of the trap period. Should also fit nicely as a factor of the DMA period.\nCompare ticks for accurate commensurability check."
        # "Oscillation frequency needs to be commensurate\nwith the data save time."
        # "Be commensurate with total save time/100 (or so). That way you are guaranteed you can average spectra at least 100x."
        n2070 = event-data() -> ()  [unwired: 7 out]
        n2071 = local read "Total Counts (ticks)"() -> (w3152:u16)
        n2072 = To Unsigned Long Integer(number=w3152) -> (unsigned 32bit integer=w3162:u32)
        n2073 = Multiply "Base osc period (ticks)"(x=w3162, y="Base N trap periods") -> (x*y=w3153:u32)
        n2074 = local read "# Samples/trap"() -> (w3157:u32)
        n2075 = Multiply "Scaled osc period (ticks)"(x=w3153, y="Period scale factor") -> (x*y=w3154:dbl)
        n2076 = Multiply(x="Base N trap periods", y="Period scale factor") -> ()  [unwired: 1 out]
        n2077 = local read "Cal sets to save"() -> (w3158:u32)
        n2078 = To Unsigned Quad Integer(1:w3154) -> (0:w3144:u64)
        n2079 = for "vector 0 to N -1" {
          N: w3130 -> [_]
          tunnel: [w3179] -> w3150 mode=indexing
          i -> [w3179]
        }
        n2080 = Multiply "Ticks/DMA"(x=w3157, y=w3162) -> (x*y=w3161:u32)
        n2081 = Multiply "Scaled osc period (s)"(x=w3144, y=2.5e-08) -> (x*y=w3156:dbl)
        "Trap OSC Period (s)" <- w3156
        n2082 = Reciprocal(x=w3156) -> (1/x=→"A cal freq (Hz)":dbl)
        n2083 = Multiply(x=w3150, y=6.283185307179586) -> (x*y=w3165:dbl[])
        n2084 = Quotient & Remainder(x=w3161, y=w3144) -> (x-y*floor(x/y)=w3137:u64, floor(x/y)=→"N osc / DMA":u64)
        "DMA remainder" <- w3137
        n2085 = Multiply "Total trap ticks"(x=w3158, y=w3161) -> (x*y=w3145:u32)
        n2086 = Divide(x=w3165, y=w3130) -> (x/y=w3166:dbl[])
        n2087 = Sine(x=w3166) -> (sin(x)=w3167:dbl[])
        n2088 = Quotient & Remainder(x=w3145, y=100) -> (x-y*floor(x/y)=w3140:u32, floor(x/y)=w3160:u32)
        "Total save/100 remainder" <- w3140
        n2089 = Multiply "Single period osc vector"(x=w3167, y="Trap osc amp (MHz)") -> (x*y=w3143:dbl[])
        n2090 = Quotient & Remainder(x=w3160, y=w3144) -> (x-y*floor(x/y)=w3139:u64, floor(x/y)=→"N osc/ (total save/100)":u64)
        "(total save/100) /osc period remainder" <- w3139
        n2091 = Quotient & Remainder(x=w3145, y=w3144) -> (x-y*floor(x/y)=w3138:u64)  [unwired: 1 out]
        "N trap osc periods per save remainder" <- w3138
        n2092 = call "IR AOM freq to word - vec.vi"("Frequency In (double vec, MHz)"=w3143) -> ("Frequency Word Out"=w3142:dbl[])
        n2093 = To Quad Integer(1:w3142) -> (0:w3141:i64[])
        n2094 = disable-structure shown="Disabled" {
          disable-tunnel: w3149 -> [w3171 _]
          disable-tunnel: w3141 -> [w3169 _]
          frame Disabled {
            n2095 = xnode "Read/Write Control"("FPGA VI Reference In"=w3171) -> ("FPGA VI Reference Out"=w3170:T35)  [unwired: 3 in, 1 out]
            n2096 = flat-sequence {
              tunnel: w3169 -> [w3174]
              tunnel: w3170 -> [w3173]
              frame #0 {
                n2097 = for "Write data to fpga memory" {
                  tunnel: w3173 -> [w3176]
                  tunnel: w3174 -> [_] mode=indexing
                  (unwired) TRUE ("Ready Write")
                  n2098 = xnode "Read/Write Control"("FPGA VI Reference In"=w3176) -> ("FPGA VI Reference Out"=w3175:T35)  [unwired: 4 in, 1 out]
                  n2099 = while {
                    tunnel: w3175 -> [w3177]
                    stop <- _ continue-if-true
                    n2100 = xnode "Read/Write Control"("FPGA VI Reference In"=w3177) -> ()  [unwired: 1 in, 3 out]
                  }
                }
                "Writing waveform to fpga memory" <- TRUE ("Writing waveform to fpga memory")
              }
              frame #1 {
                n2101 = local write "Writing waveform to fpga memory"(FALSE ("Writing waveform to fpga memory")) -> ()
              }
            }
          }
          frame Enabled {
          }
        }
        n2102 = Equal?(x=w3139, y=w3136) -> (x = y?=w3134:bool)
        n2103 = Equal?(x=w3140, y=w3136) -> (x = y?=w3135:bool)
        n2104 = Equal?(x=w3137, y=w3136) -> (x = y?=w3132:bool)
        n2105 = Equal?(x=w3138, y=w3136) -> (x = y?=w3133:bool)
        n2106 = Compound Arithmetic op=AND(w3135, w3134, w3133, w3132) -> (→"Good freq?":bool)
      }
      event "Osc trap cont.", "Osc traps", "T1 Osc Enable", "T2 Osc Enable": Value Change {
        n2107 = event-data() -> ()  [unwired: 7 out]
        n2108 = disable-structure shown="Disabled" {
          disable-tunnel: w3180 -> [w3183 _]
          frame Disabled {
            n2109 = xnode "Read/Write Control"("FPGA VI Reference In"=w3183, "Trap 1 osc enable"="T1 Osc Enable", "Trap 2 osc enable"="T2 Osc Enable") -> ()  [unwired: 1 in, 2 out]
          }
          frame Enabled {
          }
        }
      }
      event "Pressure Pump Voltage (+/-10V)": Value Change {
        n2110 = event-data() -> ()  [unwired: 7 out]
        n2111 = disable-structure shown="Disabled" {
          disable-tunnel: w3184 -> [w3188 _]
          frame Disabled {
            n2112 = Divide(x="Pressure Pump Voltage (+/-10V)", y=10.0) -> (x/y=w3185:dbl)
            n2113 = Multiply(x=w3185, y=32767.0) -> (x*y=w3186:dbl)
            n2114 = xnode "Read/Write Control"("FPGA VI Reference In"=w3188, "Pressure Pump"=w3186) -> ()  [unwired: 1 in, 2 out]
          }
          frame Enabled {
          }
        }
      }
      event "Dynamic Force FB (ronen)": Value Change {
        # "Added by ronen - for feedback on trap position by changing the actual frequency and not the set frequency - for increasing the range of feedback."
        n2115 = event-data() -> ()  [unwired: 7 out]
        n2116 = xnode "Read/Write Control"("FPGA VI Reference In"=w3192, "Dynamic Force FB (Ronen)"="Dynamic Force FB (ronen)") -> ()  [unwired: 1 in, 2 out]
      }
      event "Read Setpoint Correction File": Value Change {
        n2117 = event-data() -> ()  [unwired: 7 out]
        n2118 = local write "Read Setpoint Correction File"(FALSE ("Read Setpoint Correction File")) -> ()
        n2119 = Open/Create/Replace File(file path (use dialog)="Setpoint Correction Offset File", operation (0:open)=T43."open", access (0:read/write)=enum16{"read/write", "read-only", "write-only"}."read-only") -> (refnum out=w3216:refnum<file>)  [unwired: 1 in, 4 out]
        n2120 = Deny Access(7:w3216) -> (3:w3215:refnum<file>)  [unwired: 1 in, 2 out]
        n2121 = Read from Binary File(5:0.0, 9:T44."big-endian, network order" ("byte order (0:big-endian, network order)"), 10:-1 ("count (1)"), 11:w3215) -> (2:w3209:dbl[], 3:w3214:refnum<file>)  [unwired: 1 in, 3 out]
        n2122 = Close File(refnum=w3214) -> ()  [unwired: 1 in, 2 out]
        n2123 = Array Subset(array=w3209, index=3) -> (w3210:dbl[])  [unwired: 1 in]
        n2124 = Index Array(array=w3209, index=0) -> (element=w3198:dbl)
        n2125 = local read "T2 calibration"() -> (w3197:T8)
        n2126 = local read "T1 calibration"() -> (w3205:T9)
        n2127 = local write "Offset file step size"(w3198) -> ()
        n2128 = Unbundle By Name(w3197) -> ("T2 alpha_x (nm/V)"=w3200:dbl, "T2 kappa_x (pN/nm)"=w3199:dbl)
        n2129 = Unbundle By Name(w3205) -> ("T1 alpha_x (nm/V)"=w3202:dbl, "T1 kappa_x (pN/nm)"=w3201:dbl)
        n2130 = Multiply(x=w3202, y=w3201) -> (x*y=w3203:dbl)
        n2131 = Multiply(x=w3200, y=w3199) -> (x*y=w3204:dbl)
        n2132 = Decimate 1D Array(w3210) -> (w3207:dbl[], w3206:dbl[])  [unwired: 1 out]
        n2133 = Divide(x=w3204, y=w3203) -> (x/y=w3194:dbl)
        n2134 = property on="B factor" class="DigNum (strict)"("Val(Sgnl)"=w3194) -> ()  [unwired: 2 in, 2 out]
        n2135 = Multiply(x=w3206, y=w3194) -> (x*y=w3208:dbl[])
        n2136 = Subtract(x=w3207, y=w3208) -> (x-y=w3193:dbl[])
        n2137 = local read "Offset Values"() -> (w3196:T20)
        n2138 = Bundle By Name(cluster=w3196, "Trap 1X offset"=w3207, "Trap 2X offset"=w3206) -> (w3195:T20)
        n2139 = local write "Offset Values"(w3195) -> ()
        n2140 = property on="Setpoint offset\ncorrection values" class="Arr (strict)"("Val(Sgnl)"=w3193) -> ()  [unwired: 2 in, 2 out]
      }
      event "B factor", "Setpoint offset\ncorrection values", "Target Force (pN)": Value Change {
        w3253 = 6.0  # clock mult.
        w3254 = 49152000.0  # TCXO frequ.
        n2141 = event-data() -> ()  [unwired: 7 out]
        n2142 = local read "B factor"() -> (w3255:dbl)
        n2143 = xnode "Read/Write Control"("FPGA VI Reference In"=w3256, "B factor"=w3255) -> ("BD1 Frequency Out 1"=w3246:u64)  [unwired: 1 in, 2 out]
        n2144 = To Double Precision Float(number=w3246) -> (double precision float=w3252:dbl)
        n2145 = local read "BD 1 Frequency 2 (MHz)"() -> (w3244:dbl)
        n2146 = Multiply(x=w3254, y=w3253) -> (x*y=w3251:dbl)
        n2147 = Multiply(x=w3252, y=w3251) -> (x*y=w3250:dbl)
        n2148 = Scale By Power Of 2(n=-48, x=w3250) -> (x*2^n=w3248:dbl)
        n2149 = Divide(x=w3248, y=1000000.0) -> (x/y=w3245:dbl)
        n2150 = Subtract(x=w3244, y=w3245) -> (x-y=w3232:dbl)
        n2151 = local read "Target Force (pN)"() -> (w3243:dbl)
        n2152 = local read "T1 calibration"() -> (w3241:T9)
        n2153 = local read "Offset file step size"() -> (w3231:dbl)
        n2154 = local read "Setpoint offset\ncorrection values"() -> (w3228:dbl[])
        n2155 = Unbundle By Name(w3241) -> ("T1 alpha_x (nm/V)"=w3240:dbl, "T1 kappa_x (pN/nm)"=w3239:dbl)
        n2156 = Multiply(x=w3243, y=2.0) -> (x*y=w3237:dbl)
        n2157 = Divide(x=w3232, y=w3231) -> (x/y=w3230:dbl)
        n2158 = local read "Negate Diff?"() -> (w3234:bool)
        n2159 = To Long Integer(number=w3230) -> (32bit integer=w3229:i32)
        n2160 = Multiply(x=w3240, y=w3239) -> (x*y=w3238:dbl)
        n2161 = Index Array(array=w3228, index=w3229) -> (element=w3226:dbl)
        n2162 = Divide(x=w3237, y=w3238) -> (x/y=w3233:dbl)
        n2163 = Select(t=1, s=w3234, f=-1) -> (s? t:f=w3227:i32)
        n2164 = Multiply(x=w3227, y=w3226) -> (x*y=w3225:dbl)
        n2165 = Add(x=w3233, y=w3225) -> (x+y=w3224:dbl)
        n2166 = To Fixed-Point(number=w3224) -> (fixed-point=w3223:fxp<+/-,16,1>)  [unwired: 1 in]
        n2167 = property on="Trap Pos FB SP" class="DigNum (strict)"("Val(Sgnl)"=w3223) -> ()  [unwired: 2 in, 2 out]
      }
      event "Trap 3 (ON/OFF)", "T3 Y (V)", "T3 X (V)": Value Change {
        n2168 = event-data() -> ()  [unwired: 7 out]
        n2169 = case shown="False" "Trap 3 (ON/OFF)" {
          tunnel: [5.0 0.0] -> w3258
          frame False {
          }
          frame True {
          }
        }
        n2170 = Multiply(x="T3 X (V)", y=32767.0) -> (x*y=w3274:dbl)
        n2171 = Multiply(x="T3 Y (V)", y=32767.0) -> (x*y=w3271:dbl)
        n2172 = Divide(x=w3274, y=10.0) -> (x/y=w3275:dbl)
        n2173 = Divide(x=w3271, y=10.0) -> (x/y=w3270:dbl)
        n2174 = To Unsigned Word Integer(number=w3275) -> (unsigned 16bit integer=w3264:u16)
        n2175 = To Unsigned Word Integer(number=w3270) -> (unsigned 16bit integer=w3265:u16)
        n2176 = Multiply(x=w3258, y=32767.0) -> (x*y=w3261:dbl)
        n2177 = Divide(x=w3261, y=10.0) -> (x/y=w3260:dbl)
        n2178 = To Unsigned Word Integer(number=w3260) -> (unsigned 16bit integer=w3257:u16)
        n2179 = xnode "Read/Write Control"("FPGA VI Reference In"=w3266, "Piezo Trap X (AO5)"=w3264, "Piezo Trap Y (AO4)"=w3265, "Piezo Trap ON/Off (AO3)"=w3257) -> ()  [unwired: 1 in, 2 out]
      }
      event "Cursor control.X", "Cursor control.Y": Value Change {
        # "If turning cursor control off, update the piezo controls"
        n2180 = event-data() -> ()  [unwired: 7 out]
        n2181 = xnode "Read/Write Control"("FPGA VI Reference In"=w3285) -> ("Piezo X out"=w3283:u16, "Piezo Y out"=w3279:u16)  [unwired: 1 in, 2 out]
        n2182 = local read "Cursor control"() -> (w3284:cluster{"X":bool, "Y":bool})
        n2183 = Unbundle By Name(w3284) -> ("X"=w3282:bool, "Y"=w3281:bool)
        n2184 = And(x=w3282, y=w3281) -> (x .and. y?=w3280:bool)
        n2185 = case shown="True" w3280 {
          tunnel: w3283 -> [w3290 _]
          tunnel: w3279 -> [w3288 _]
          frame False {
            w3287 = 3276.7
            n2186 = Divide(x=w3290, y=w3287) -> (x/y=w3289:dbl)
            n2187 = Divide(x=w3288, y=w3287) -> (x/y=w3286:dbl)
            n2188 = property on="T3 X (V)" class="DigNum (strict)"("Val(Sgnl)"=w3289) -> ()  [unwired: 2 in, 2 out]
            n2189 = property on="T3 Y (V)" class="DigNum (strict)"("Val(Sgnl)"=w3286) -> ()  [unwired: 2 in, 2 out]
          }
          frame True {
          }
        }
      }
    }
    "error out 2" <- w1671
    n2190 = node-c288() -> ()  [unwired: 2 out]
  }
  n2191 = node-c288() -> (w64:T36)  [unwired: 4 out]
  n2192 = timed-loop "Mouse control: trap position (AOM deflection), set confocal spot from image" {
    tunnel: [w3291] -> w69
    timing: w64 -> [_]
    timing-out: [_] -> w63
    tunnel: w21 -> [w3292]
    stop <- w3291 stop-if-true
    n2193 = node-c288() -> ()  [unwired: 2 out]
    n2194 = event shown="[0] \"Pane\": Mouse Down" {
      selector: _ -> [_ _ _ _]
      dyn-events: _ -> [_ _ _ _]
      timeout: _ -> [_ _ _ _]
      tunnel: w3292 -> [w3295 _ _ _]
      tunnel: [_ _ TRUE _] -> w3291
      event Mouse Down {
        n2195 = event-data() -> ("Time"=w3297:u32, "Coords"=w3296:T12, "Button"=w3298:u16)  [unwired: 6 out]
        n2196 = case shown="1" w3298 {
          tunnel: w3297 -> [_ _ w3404]
          tunnel: w3296 -> [_ w3335 w3402]
          tunnel: w3295 -> [_ _ w3398]
          frame 0, Default {
          }
          frame 1 {
            n2197 = property on="APD 2" class="ImageControl"() -> ("Displayed Image Position"=w3305:cluster{"Left":i32, "Top":i32})  [unwired: 2 in, 2 out]
            n2198 = property on="APD 1" class="ImageControl"() -> ("Displayed Image Position"=w3334:cluster{"Left":i32, "Top":i32})  [unwired: 2 in, 2 out]
            n2199 = property on="Detection Laser X" class="ImageControl"() -> ("Displayed Image Position"=w3331:cluster{"Left":i32, "Top":i32})  [unwired: 2 in, 2 out]
            n2200 = property on="Detection Laser Y" class="ImageControl"() -> ("Displayed Image Position"=w3330:cluster{"Left":i32, "Top":i32})  [unwired: 2 in, 2 out]
            n2201 = property on="APD 2" class="ImageControl"() -> ("Displayed Image Size"=w3304:cluster{"Width":u32, "Height":u32})  [unwired: 2 in, 2 out]
            n2202 = property on="APD 1" class="ImageControl"() -> ("Displayed Image Size"=w3332:cluster{"Width":u32, "Height":u32})  [unwired: 2 in, 2 out]
            n2203 = property on="Detection Laser X" class="ImageControl"() -> ("Displayed Image Size"=w3333:cluster{"Width":u32, "Height":u32})  [unwired: 2 in, 2 out]
            n2204 = property on="Detection Laser Y" class="ImageControl"() -> ("Displayed Image Size"=w3329:cluster{"Width":u32, "Height":u32})  [unwired: 2 in, 2 out]
            n2205 = Unbundle By Name(w3304) -> ("Width"=w3301:u32, "Height"=w3300:u32)
            n2206 = Unbundle By Name(w3305) -> ("Left"=w3303:i32, "Top"=w3302:i32)
            n2207 = Unbundle By Name(w3332) -> ("Width"=w3326:u32, "Height"=w3325:u32)
            n2208 = Unbundle By Name(w3333) -> ("Width"=w3322:u32, "Height"=w3321:u32)
            n2209 = Unbundle By Name(w3329) -> ("Width"=w3318:u32, "Height"=w3317:u32)
            n2210 = Unbundle By Name(w3334) -> ("Left"=w3328:i32, "Top"=w3327:i32)
            n2211 = Unbundle By Name(w3331) -> ("Left"=w3324:i32, "Top"=w3323:i32)
            n2212 = Unbundle By Name(w3330) -> ("Left"=w3320:i32, "Top"=w3319:i32)
            n2213 = Bundle("Left"=w3303, "Top"=w3302, "Width"=w3301, "Height"=w3300) -> (w3299:T48)  [unwired: 1 in]
            n2214 = Bundle("Left"=w3328, "Top"=w3327, "Width"=w3326, "Height"=w3325) -> (w3316:T48)  [unwired: 1 in]
            n2215 = Bundle("Left"=w3324, "Top"=w3323, "Width"=w3322, "Height"=w3321) -> (w3315:T48)  [unwired: 1 in]
            n2216 = Bundle("Left"=w3320, "Top"=w3319, "Width"=w3318, "Height"=w3317) -> (w3314:T48)  [unwired: 1 in]
            n2217 = Build Cluster Array(w3299, w3316, w3315, w3314) -> (w3313:T49)
            n2218 = for {
              tunnel: w3335 -> [w3346]
              tunnel: w3313 -> [w3347] mode=indexing
              shift-right: [w3344] -> w3311
              shift-left: TRUE -> [w3345]
              shift-right: [w3343] -> w3309
              shift-left: _ -> [w3339]
              shift-right: [w3342] -> w3308
              shift-left: _ -> [w3338]
              shift-right: [w3341] -> w3307
              shift-left: _ -> [w3337]
              shift-right: [w3340] -> w3306
              shift-left: _ -> [w3336]
              n2219 = case shown="True" w3345 {
                selector: w3345 -> [w3352 _]
                tunnel: w3347 -> [_ w3361]
                tunnel: w3346 -> [_ w3359]
                tunnel: [w3352 w3357] -> w3344
                tunnel: [w3351 w3356] -> w3343
                tunnel: [w3350 w3355] -> w3342
                tunnel: [w3349 w3354] -> w3341
                tunnel: [w3348 w3353] -> w3340
                tunnel: w3339 -> [w3351 _]
                tunnel: w3338 -> [w3350 _]
                tunnel: w3337 -> [w3349 _]
                tunnel: w3336 -> [w3348 _]
                frame False {
                }
                frame True {
                  n2220 = Unbundle(w3361) -> (w3360:T48)
                  n2221 = call "isclickinwindow.vi"("Image Param"=w3360, "Point32"=w3359) -> ("4 Y"=w3353:i32, "3 Height"=w3354:i32, "2 X"=w3355:i32, "1 Width"=w3356:i32, "In image?"=w3358:bool)  [unwired: 1 in]
                  n2222 = Not(x=w3358) -> (.not. x?=w3357:bool)
                }
              }
            }
            n2223 = Not(x=w3311) -> (.not. x?=w3310:bool)
            n2224 = case shown="True" w3310 {
              tunnel: w3308 -> [_ w3375]
              tunnel: w3306 -> [_ w3374]
              tunnel: w3309 -> [_ w3373]
              tunnel: w3307 -> [_ w3372]
              frame False {
              }
              frame True {
                w3362 = FALSE ("Get Point")
                n2225 = local read "Scan lines (y)"() -> (w3377:u64)
                n2226 = disable-structure shown="Disabled" {
                  frame Disabled {
                  }
